vi "AlazarSetTriggerOperation.vi"(0 "Handle":u32, 1 "Operation":u32(ring) items=["J", "K", "J OR K", "J AND K", "J XOR K", "J AND NOT K", "NOT J AND K"], 5 "error in (no error)":errorcluster, 6 "Engine X":u32(ring) items=["J", "K"], 7 "Engine Y":u32(ring)=1 items=["J", "K"], 8 "X Source":u32(ring) items=["A", "B", "External", "Disable", "C", "D"], 9 "Y Source":u32(ring)=3 items=["A", "B", "External", "Disable", "C", "D"], 10 "X Slope":u32(ring)=1 items=["Positive"=1, "Negative"=2], 11 "Y Slope":u32(ring)=1 items=["Positive"=1, "Negative"=2], 12 "X Level":u32, 13 "Y Level":u32) -> (14 "Handle":u32, 18 "Return Code":u32, 19 "error out":errorcluster)   [LabVIEW 2021]
doc: "Configure the trigger system."
uses:
  ATSApi.dll
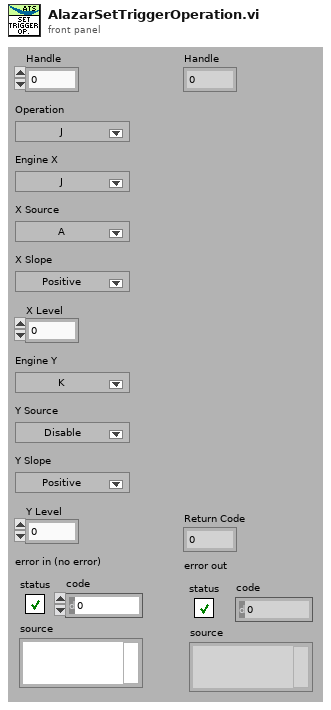
[diagram p1: front panel]
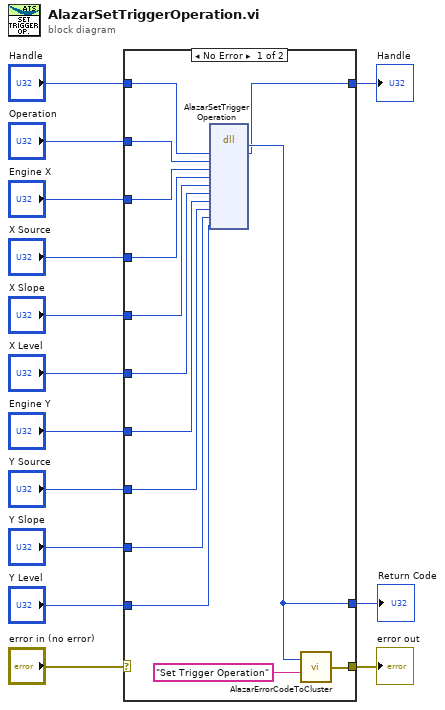
[diagram p0: block diagram]
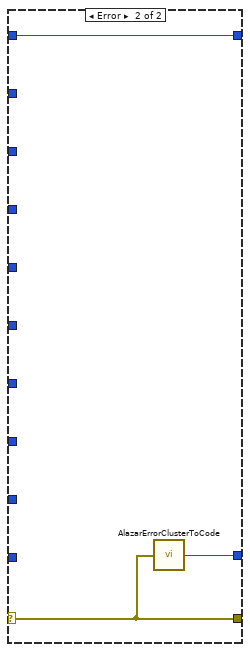
[diagram p2: hidden frame]
diagram:
  n1 = case shown="No Error" "error in (no error)" {
    selector: "error in (no error)" -> [_ w31]
    tunnel: [w25 w31] -> w13
    tunnel: [w27 w30] -> w12
    tunnel: "Handle" -> [w28 w29]
    tunnel: [w24 w29] -> w10
    tunnel: "Operation" -> [w23 _]
    tunnel: "Engine X" -> [w22 _]
    tunnel: "X Source" -> [w21 _]
    tunnel: "X Slope" -> [w20 _]
    tunnel: "X Level" -> [w19 _]
    tunnel: "Engine Y" -> [w18 _]
    tunnel: "Y Source" -> [w17 _]
    tunnel: "Y Slope" -> [w16 _]
    tunnel: "Y Level" -> [w15 _]
    frame No Error {
      n2 = dll-call lib="ATSApi.dll" fn="AlazarSetTriggerOperation"("handle"=w28, "triggerOperation"=w23, "triggerEngine1"=w22, "source1"=w21, "slope1"=w20, "level1"=w19, "triggerEngine2"=w18, "source2"=w17, "slope2"=w16, "level2"=w15) -> (w27:u32, "handle"=w24:u32)  [unwired: 12 in, 2 out]
      n3 = call "AlazarErrorCodeToCluster.vi"("Message"="Set Trigger Operation", "Error Code"=w27) -> ("error out"=w25:errorcluster)
    }
    frame Error {
      n4 = call "AlazarErrorClusterToCode.vi"("error in (no error)"=w31) -> ("Error Code"=w30:u32)
    }
  }
  "Handle" <- w10
  "error out" <- w13
  "Return Code" <- w12
